vi "count letters.vi"(8 "error in (no error)":errorcluster, 11 "Integer written in English":string) -> (0 "error out":errorcluster, 3 "no. of letters":i32)   [LabVIEW 2021, in "Project Euler.lvlib"]
uses:
  Project Euler.lvlib
  <userlib>/_OpenG.lib/array/array.llb/Filter 1D Array (String)__ogtk.vi
panel:
  # "Development\ncontrols/indicators useful for development and testing, but which are not outputs of the VI"
  # "Input\nInputs to the VI"
  # "Output\nOutputs of the VI"
  # "Description\n\nBlank VI with error handling case. \n\nSummarize the use of this VI in this space."
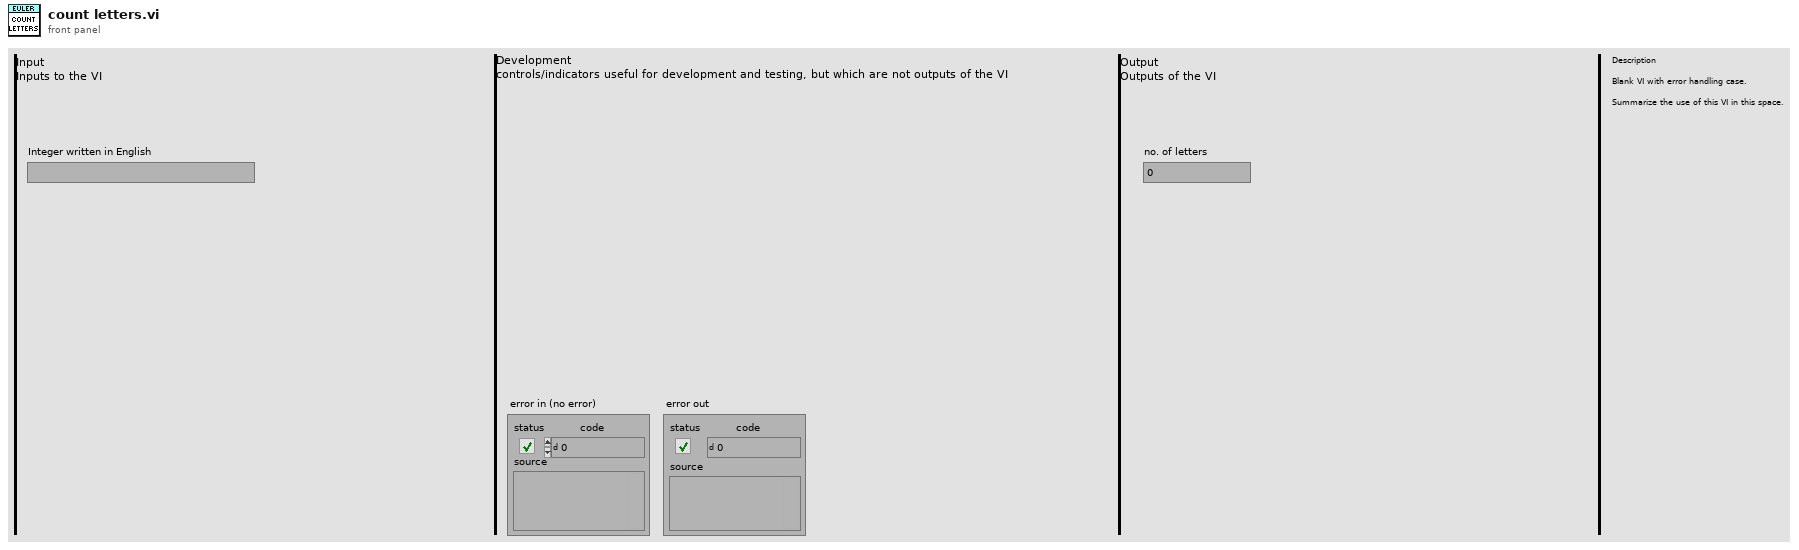
[diagram p1: front panel]
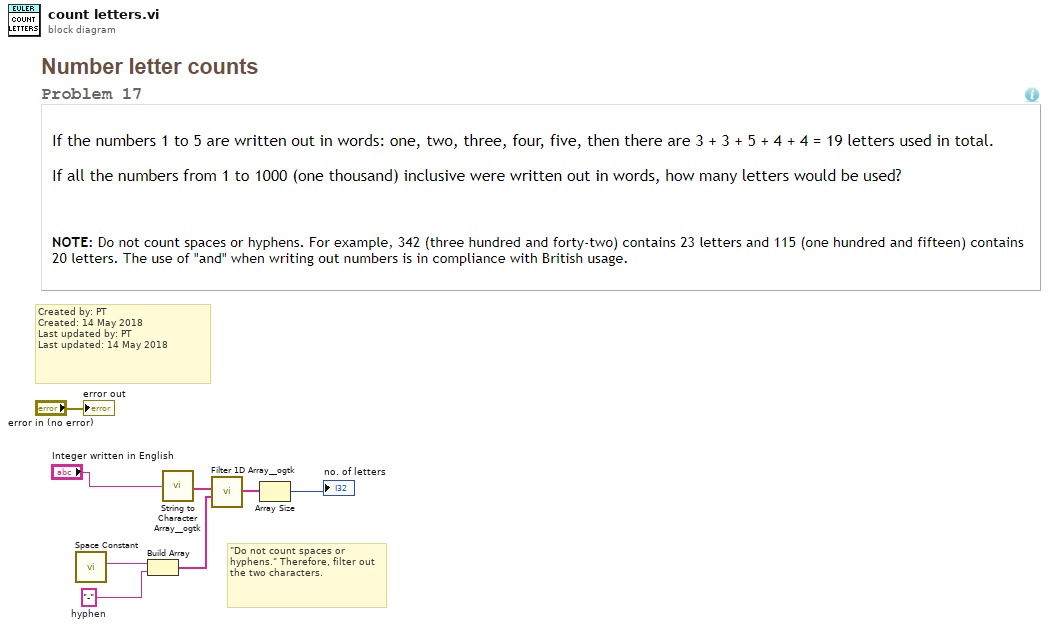
[diagram p0: block diagram]
diagram:
  w4 = "-"  # hyphen
  # "\"Do not count spaces or hyphens.\" Therefore, filter out the two characters."
  # "Created by: PT\nCreated: 14 May 2018\nLast updated by: PT\nLast updated: 14 May 2018"
  n1 = call <vilib>:"Space Constant.vi"() -> ("String"=w5:string)
  n2 = Build Array(w5, w4) -> (w3:string[])
  n3 = call <userlib>:"String to Character Array__ogtk.vi"("Input String"="Integer written in English") -> ("Character Array"=w6:string[])
  n4 = call-poly <userlib>:"Filter 1D Array__ogtk.vi"("items to filter"=w3, "array"=w6) -> ("filtered array"=w2:string[])  [unwired: 4 in, 1 out]
  n5 = Array Size(array=w2) -> (size(s)=→"no. of letters":i32)
  "error out" <- "error in (no error)"
